vi "Configure Reference.vi"(0 "VISA resource name":refnum<visa-resource-name>, 1 "Scan List (Empty)":string, 5 "Reference Method (0: Off)":u16(ring) items=["Off", "Manual", "Acquire"], 7 "Reference Value (0)":dbl, 11 "error in (no error)":errorcluster) -> (4 "VISA resource name out":refnum<visa-resource-name>, 15 "error out":errorcluster)   [LabVIEW 2020, in "Keithley 27XX.lvlib"]
doc: "This VI configures the Reference attributes used in relative functions. The relative function can be used to null offsets or subtract a baseline reading from present and future readings. When enabled, the instrument uses the present reading as a relative value. Subsequent readings will be the difference between the actual input value and the relative value.\n\nYou can define a relative value for each funciton. Once a relative value is established for a measurement fucntion, the value is the same for all ranges. For example, if 50V is set as a relative value on the 100V range, the relative value is also 50V on the 1000V, 10V, 1V and 100mV ranges.\n\nNote: \n(1) Configure Measurement.vi must be called <B>before</B> setting the reference.\n\n(2) This VI should not be used with the function \"Continuity\""
uses:
  Keithley 27XX.lvlib
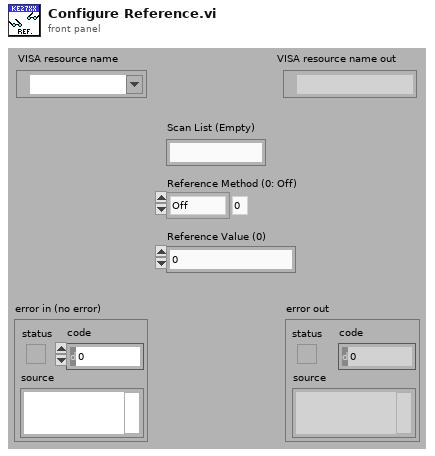
[diagram p1: front panel]
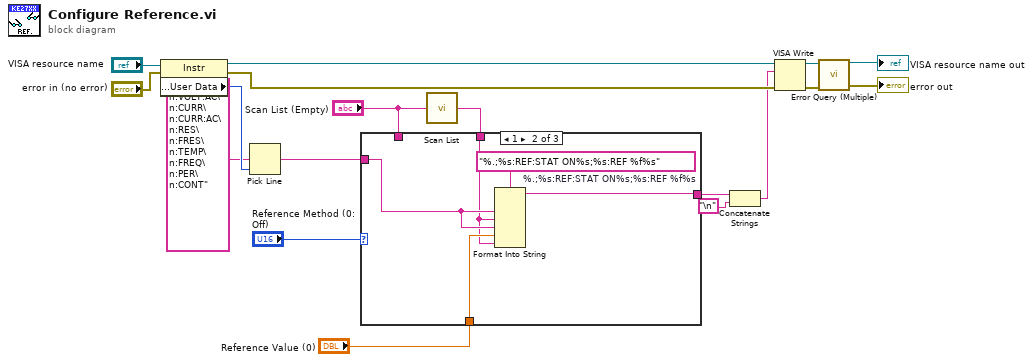
[diagram p0: block diagram]
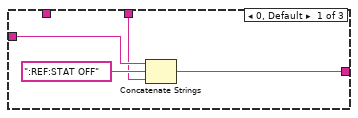
[diagram p2: hidden frame]
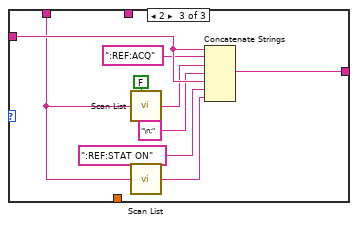
[diagram p3: hidden frame]
diagram:
  n1 = property on="Property Node" class="Instr"(reference="VISA resource name", error in="error in (no error)") -> (reference out=w12:refnum<visa-resource-name>, error out=w11:errorcluster, "General Settings:User Data"=w18:u32)
  n2 = Pick Line(multi-line string=":VOLT\n:VOLT:AC\n:CURR\n:CURR:AC\n:RES\n:FRES\n:TEMP\n:FREQ\n:PER\n:CONT", line index=w18) -> (output string=w13:string)  [unwired: 1 in]
  n3 = call "Scan List.vi"("Scan List (Empty)"="Scan List (Empty)") -> ("Scan List Out"=w1:string)  [unwired: 14 in]
  n4 = case shown="1" "Reference Method (0: Off)" {
    tunnel: [w21 w24 w36] -> w4
    tunnel: w13 -> [w20 w25 w35]
    tunnel: "Reference Value (0)" -> [_ w26 _]
    tunnel: "Scan List (Empty)" -> [_ _ w30]
    tunnel: w1 -> [w19 w23 _]
    frame 0, Default {
      n5 = Concatenate Strings(w20, ":REF:STAT OFF", w19) -> (w21:string)
    }
    frame 1 {
      w27 = "%.;%s:REF:STAT ON%s;%s:REF %f%s"  # %.;%s:REF:STAT ON%s;%s:REF %f%s
      n6 = Format Into String(format string=w27, w25, w23, w25, w26, w23) -> (resulting string=w24:string)  [unwired: 2 in, 1 out]
    }
    frame 2 {
      n7 = call "Scan List.vi"("Add Comma (True)"=FALSE, "Scan List (Empty)"=w30) -> ("Scan List Out"=w28:string)  [unwired: 13 in]
      n8 = call "Scan List.vi"("Scan List (Empty)"=w30) -> ("Scan List Out"=w29:string)  [unwired: 14 in]
      n9 = Concatenate Strings(w35, ":REF:ACQ", w28, "\n;" ("string"), w35, ":REF:STAT ON", w29) -> (w36:string)
    }
  }
  n10 = Concatenate Strings(w4, "\n") -> (w3:string)
  n11 = VISA Write(VISA resource name=w12, write buffer=w3, error in (no error)=w11) -> (VISA resource name out=w8:refnum<visa-resource-name>, error out=w9:errorcluster)  [unwired: 1 out]
  n12 = call "Error Query (Multiple).vi"("VISA resource name"=w8, "error in (no error)"=w9) -> ("VISA resource name out"=→"VISA resource name out":refnum<visa-resource-name>, "error out"=→"error out":errorcluster)  [unwired: 10 in, 2 out]
